vi "force_control_friction_frequencySwitch.vi"() -> ()   [LabVIEW 2014]
uses:
  <vilib>/rvi/interface/nirviOpenFPGA/nirviOpenFPGA.xnode
  <vilib>/rvi/interface/nirviReadWriteControl/nirviReadWriteControl.xnode
  <vilib>/rvi/interface/nirviCloseFPGA/nirviCloseFPGA.xnode
  <vilib>/rvi/Analysis/host/Public/NI_FpgaMspHost.lvlib
  FPGA Bitfiles/forceControl_FPGATarget_openloopfriction_SkQqBKVZ5ok.lvbitx
  FPGA VIs/openloop_frictiontest_Pitch.vi
panel:
  in  "frequency (Hz)":dbl format="%#_6p"
  in  "stop":bool
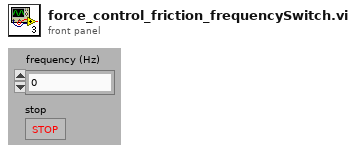
[diagram p1: front panel]
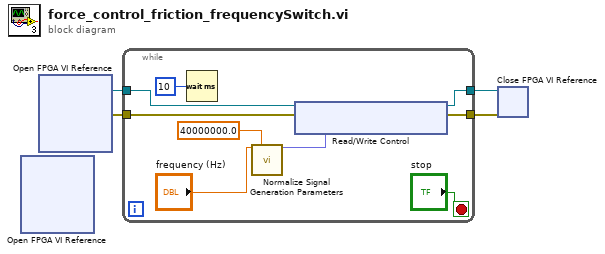
[diagram p0: block diagram]
diagram:
  n1 = xnode "Open FPGA VI Reference"() -> ()  [unwired: 2 in, 2 out]
  n2 = xnode "Open FPGA VI Reference"() -> ("FPGA VI Reference Out"=w4:refnum<k20>, "error out"=w3:errorcluster)  [unwired: 2 in]
  n3 = while {
    tunnel: w4 -> [w13]
    tunnel: w3 -> [w12]
    tunnel: [w10] -> w2
    tunnel: [w9] -> w1
    stop <- "stop" stop-if-true
    n4 = Wait (ms)(milliseconds to wait=u32 10) -> ()  [unwired: 1 out]
    n5 = call <vilib>:"Normalize Signal Generation Parameters.vi"("frequency (Hz)"="frequency (Hz)", "FPGA clock rate (Hz)"=40000000.0) -> ("frequency (periods/tick)"=w6:fxp<+,32,0>)  [unwired: 8 in, 5 out]
    n6 = xnode "Read/Write Control"("FPGA VI Reference In"=w13, "error in"=w12, "frequency (periods/tick)"=w6) -> ("FPGA VI Reference Out"=w10:refnum<k20>, "error out"=w9:errorcluster)
  }
  n7 = xnode "Close FPGA VI Reference"("FPGA VI Reference In"=w2, "error in"=w1) -> ()  [unwired: 1 out]
